vi "Handle Events.vi"(8 "error in (no error)":errorcluster, 11 "EventHandler":refnum<class "IEventHandler.lvclass">) -> ()   [LabVIEW 2020, in "ActorEvents.lvlib" / "IEventHandler.lvclass"]
doc: "处理事件"
uses:
  IEventHandler.lvclass
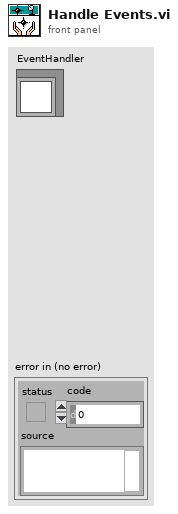
[diagram p1: front panel]
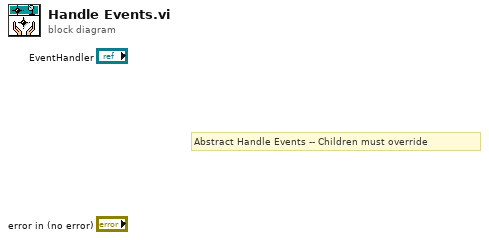
[diagram p0: block diagram]
diagram:
  # "Abstract Handle Events -- Children must override"
